vi "Polyphase Filter.vi"   [LabVIEW 2017, in "NI_AAL_Filter.lvlib"]
doc: "Filters a signal continuously with a multirate filter."
uses:
  <vilib>/Analysis/NI_AAL_Filter.lvlib
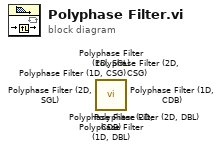
[diagram p0: block diagram]
diagram:
  n1 = call <vilib>:"Polyphase Filter (2D, CDB).vi"() -> ()  [unwired: 10 in, 2 out]
  n2 = call <vilib>:"Polyphase Filter (2D, CSG).vi"() -> ()  [unwired: 10 in, 2 out]
  n3 = call <vilib>:"Polyphase Filter (2D, SGL).vi"() -> ()  [unwired: 10 in, 2 out]
  n4 = call <vilib>:"Polyphase Filter (1D, CDB).vi"() -> ()  [unwired: 10 in, 2 out]
  n5 = call <vilib>:"Polyphase Filter (1D, CSG).vi"() -> ()  [unwired: 10 in, 2 out]
  n6 = call <vilib>:"Polyphase Filter (1D, SGL).vi"() -> ()  [unwired: 10 in, 2 out]
  n7 = call <vilib>:"Polyphase Filter (2D, DBL).vi"() -> ()  [unwired: 10 in, 2 out]
  n8 = call <vilib>:"Polyphase Filter (1D, DBL).vi"() -> ()  [unwired: 10 in, 2 out]
